vi "ArrayFuncUses.vi"() -> ()   [LabVIEW 2019]
uses:
  aa98bb20-66f4-4400-b25b-0862bfb30ec0.vi
panel:
  out "array (last n elements first)":dbl[](array[numeric])
  out "index of element":i32
  out "array with duplicates removed":dbl[](array[numeric])
  out "reversed array":dbl[](array[numeric])
  out "sorted array":dbl[](array[numeric])
  out "min value":dbl
  out "max value":dbl
  out "appended array":dbl[][](array[numeric])
  out "size(s)":i32
  in  "Array":dbl[](array[numeric])
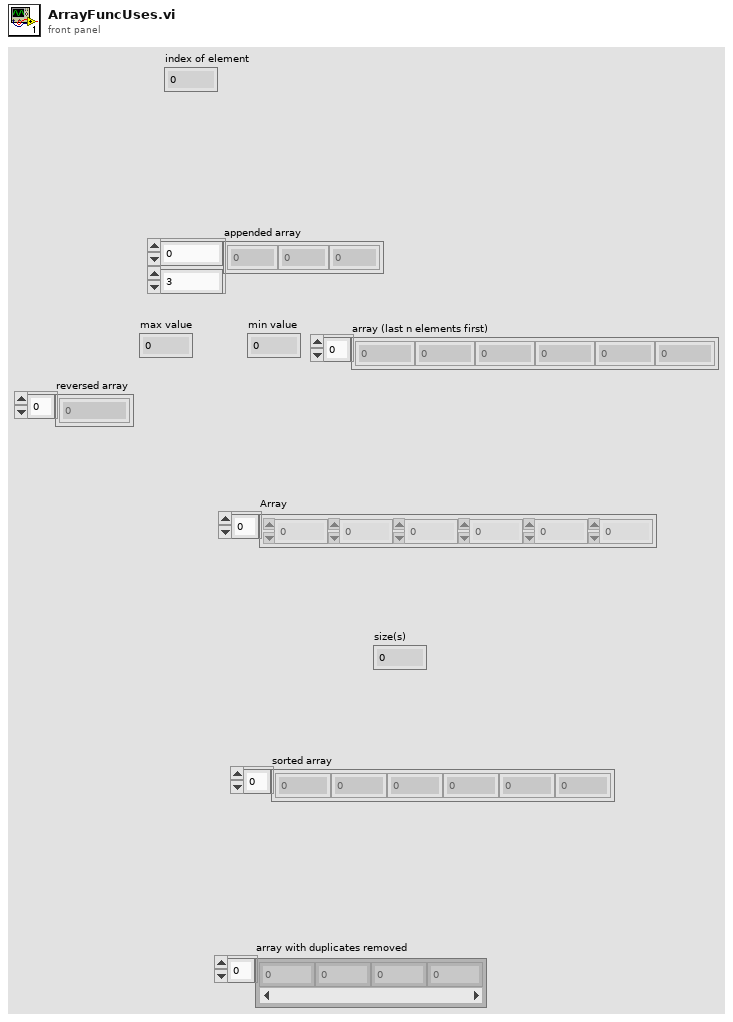
[diagram p1: front panel]
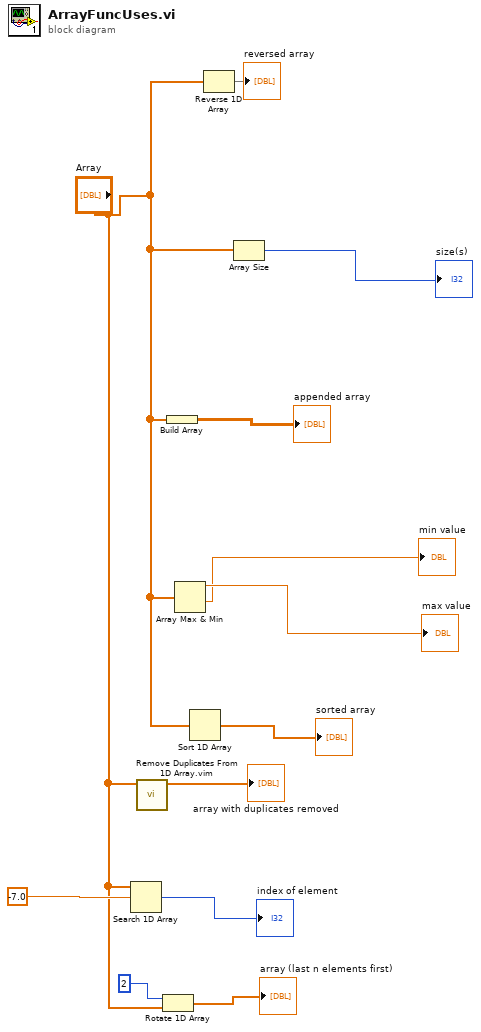
[diagram p0: block diagram]
diagram:
  n1 = Search 1D Array(1D array="Array", element=-7.0) -> (index of element=→"index of element":i32)  [unwired: 1 in]
  n2 = call "Remove Duplicates From 1D Array.vim"("array"="Array") -> ("array with duplicates removed"=→"array with duplicates removed":dbl[])  [unwired: 10 in]
  n3 = Rotate 1D Array(1:"Array", 2:2 ("n")) -> (0:→"array (last n elements first)":dbl[])
  n4 = Build Array("Array") -> (→"appended array":dbl[][])
  n5 = Array Max & Min(array="Array") -> (max value=→"max value":dbl, min value=→"min value":dbl)  [unwired: 2 out]
  n6 = Sort 1D Array(array="Array") -> (sorted array=→"sorted array":dbl[])
  n7 = Reverse 1D Array(array="Array") -> (reversed array=→"reversed array":dbl[])
  n8 = Array Size(array="Array") -> (size(s)=→"size(s)":i32)
